vi "rqcBob Alice PM Level Test (Low Level Example).vi"() -> ()   [LabVIEW 2016]
uses:
  FPGA/rqcBob/Custom Controls/Pulse Train/rqcBob Pulse Train Config.ctl
  FPGA/rqcBob/Custom Controls/Pulse Train/rqcBob Pulse Train.Generation Mode.ctl
  FPGA/rqcBob/Custom Controls/Pulse Train/rqcBob Pulse Train.First Pulse Delay Mode.ctl
  FPGA/rqcBob/Custom Controls/rqcBob Window Config.ctl
  Shared/Shared FPGA Lib/Shared Logic/Custom Controls/rqc Random Generator.parameters.ctl
  Shared/Shared FPGA Lib/Shared Logic/Custom Controls/rqc Random Generator.value type.ctl
  FPGA/rqcBob/Custom Controls/rqcBob Modulator Config.ctl
  Custom Controls/rqcBob States.ctl
  FPGA/rqcBob/Custom Controls/rqcBob Trigger Type.ctl
  Shared/Shared Host Lib/rqc ServiceNET/Custom Controls/rqc ServiceNET command.ctl
  Shared/Shared Host Lib/rqc ServiceNET/Bob/Custom Controls/rqcBob ServiceNET control.ctl
  <vilib>/FPGAPlugInAG/PCIe-7841R/niLvFpga_Open_PCIe-7841R.vi
  <vilib>/rvi/interface/common/dynamic/niFpgaDynamicAddResources.vi
  Low Level API/Configuration/Photon Detector/Detection FIFOs config/rqcBob Configure PD Detect FIFO (1PD PD1).vi
  Low Level API/Configuration/Photon Detector/Set PD window/rqcBob Configure SPD Detection Window (1PD PD1).vi
  Low Level API/Read/Read PD Detection FIFO/rqcBob Read PD Detection FIFO (1PD PD1).vi
  Shared/Shared Host Lib/rqc ServiceNET/Bob/rqcBob Send Data/rqcBob ServiceNET Send Data U32.vi
  <vilib>/FPGAPlugInAG/Dynamic/niLvFpga_Close_Dynamic.vi
  <vilib>/rvi/interface/nirviOpenFPGA/nirviOpenFPGA.xnode
  FPGA Bitfiles/rqcBob (FPGA) 7841 v 2.1.0.lvbitx
  <vilib>/rvi/interface/nirviCloseFPGA/nirviCloseFPGA.xnode
panel:
  in  "modulator.clock delay":fxp<+,4,4>
  out "current States":T1=enum."App.Stop"
  out "error out":errorcluster
  out "Connected to Alice":bool
  in  "Stop":bool
  in  "modulator.config":T2={"modulator.start"=1200, "modulator.stop"=1500}
  in  "PD.detection window":u8=11
  in  "rndGen.parameters":T3={"value type"=enum."constant", "constant"=0, "num of levels"=0, "levels values"=[0, 0, 0, 0]}
  in  "window.config":T5={"window.open"=1340, "window.close"=1640}
  in  "train.configuration":T6={"train.period"=2000, "train.num of pulses"=300, "train.mode"=enum."train sequence.single", "train.num of trains"=2000, "train.first pulse delay mode"=enum."every train", "train.first pulse delay"=55}
  in  "Port:":u16=5020
  in  "Alice's IP address":string="192.168.0.228"
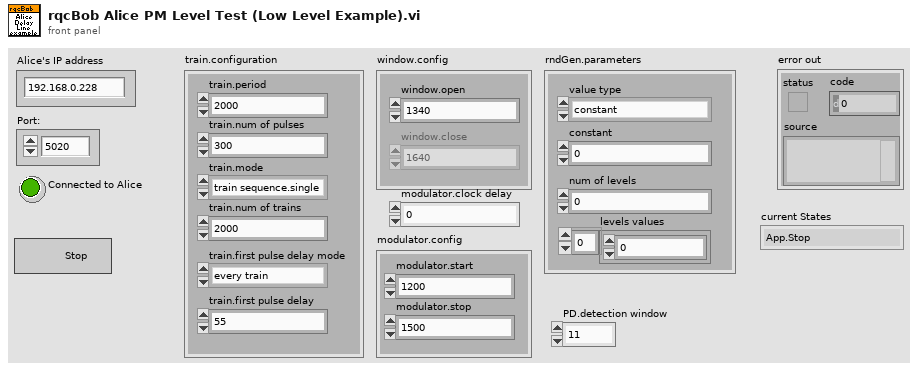
[diagram p1: front panel]
types:
  T1 = typedef "rqcBob States.ctl" = enum16{"HW.configure", "HW.sendTrigger", "HW.initiate", "HW.measure", "HW.stop", "NET.create", "NET.connect", "NET.sendCommand", "NET.readCommand", "NET.readData", "NET.close", "App.HandleEvent", "App.HandleError", "App.Stop"}
  T2 = typedef "rqcBob Modulator Config.ctl" = cluster{"modulator.start":u16, "modulator.stop":u16}
  T3 = typedef "rqc Random Generator.parameters.ctl" = cluster{"value type":T4, "constant":u16, "num of levels":u16, "levels values":u16[]}
  T4 = typedef "rqc Random Generator.value type.ctl" = enum16{"random value", "constant"}
  T5 = typedef "rqcBob Window Config.ctl" = cluster{"window.open":u16, "window.close":u16}
  T6 = typedef "rqcBob Pulse Train Config.ctl" = cluster{"train.period":u16, "train.num of pulses":u16, "train.mode":T7, "train.num of trains":u16, "train.first pulse delay mode":T8, "train.first pulse delay":u16}
  T7 = typedef "rqcBob Pulse Train.Generation Mode.ctl" = enum8{"single train", "train sequence.single", "train sequence.wait for trigger", "continuous"}
  T8 = typedef "rqcBob Pulse Train.First Pulse Delay Mode.ctl" = enum8{"none", "every train", "first train"}
  T9 = typedef "rqcBob Trigger Type.ctl" = enum16{"software", "immediate", "DIO"}
  T10 = typedef "rqc ServiceNET command.ctl" = enum8{"NONE", "READY", "START", "PING"}
  T11 = typedef "rqcBob ServiceNET control.ctl" = cluster{"connection ID":refnum<k5>, "connected?":bool, "Alice's IP address":string, "port":u16}
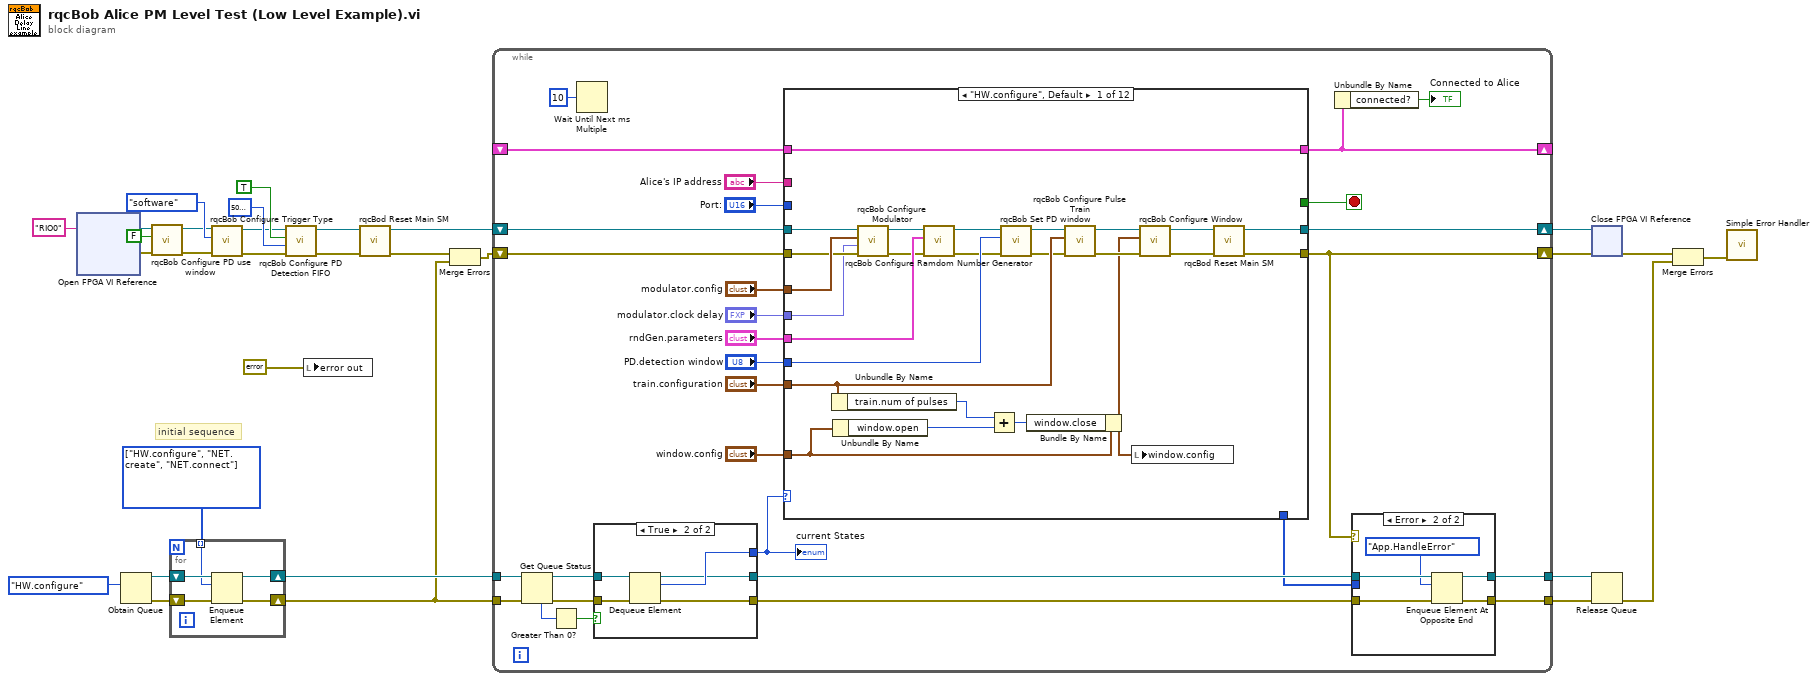
[diagram p0: block diagram]
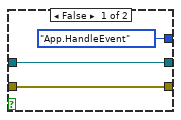
[diagram p2: hidden frame]
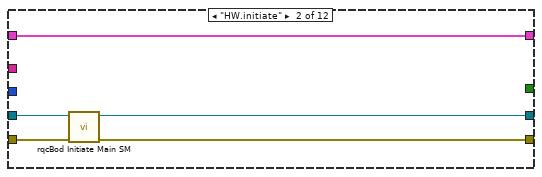
[diagram p3: hidden frame]
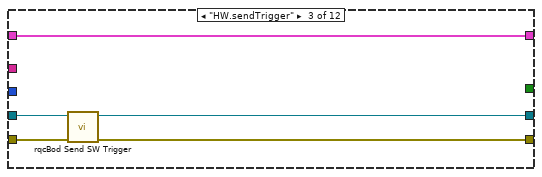
[diagram p4: hidden frame]
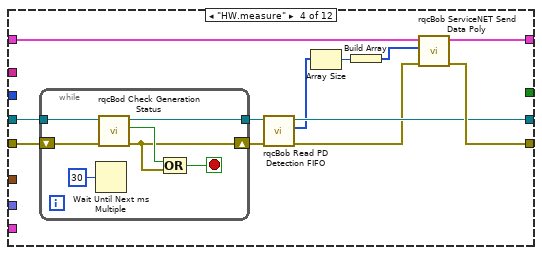
[diagram p5: hidden frame]
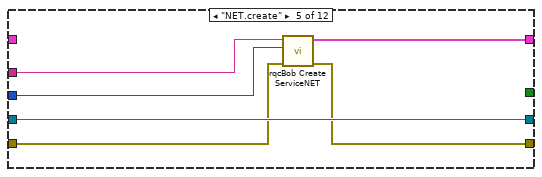
[diagram p6: hidden frame]
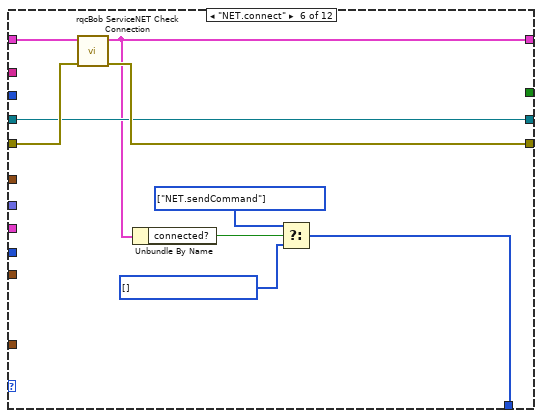
[diagram p7: hidden frame]
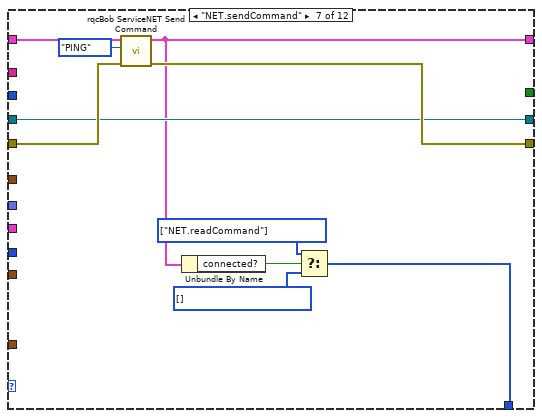
[diagram p8: hidden frame]
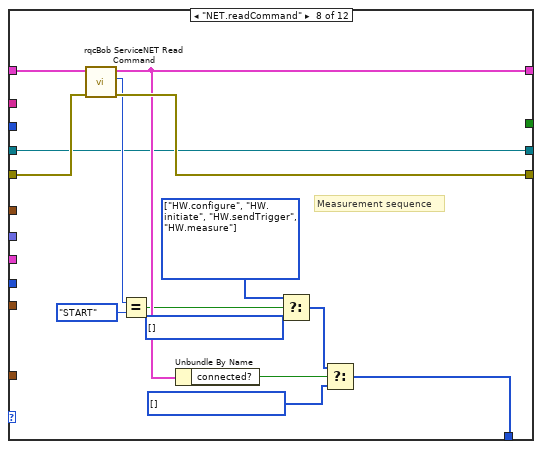
[diagram p9: hidden frame]
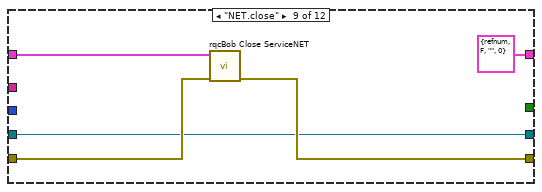
[diagram p10: hidden frame]
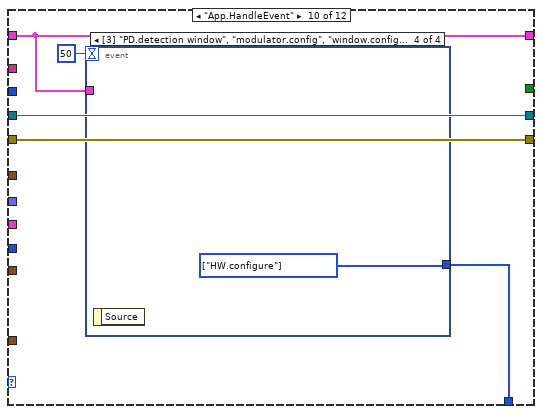
[diagram p11: hidden frame]
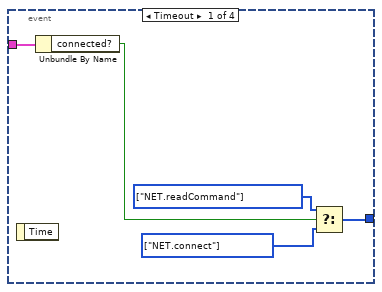
[diagram p12: hidden frame]
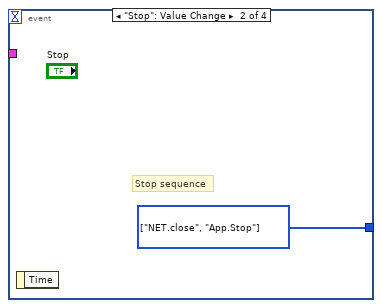
[diagram p13: hidden frame]
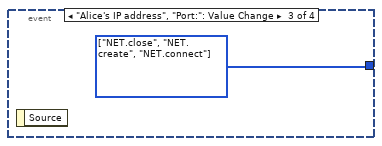
[diagram p14: hidden frame]
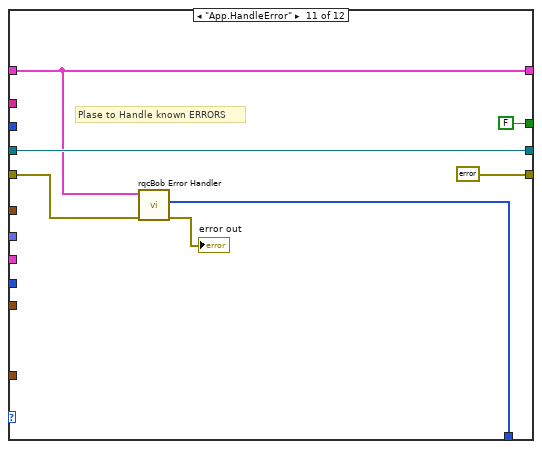
[diagram p15: hidden frame]
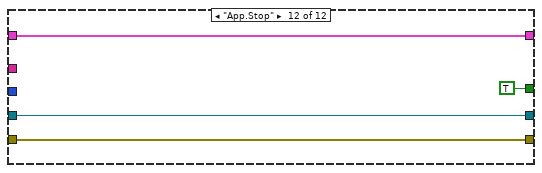
[diagram p16: hidden frame]
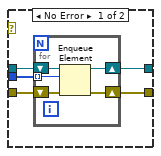
[diagram p17: hidden frame]
diagram:
  w21 = T1[] [enum."HW.configure", enum."NET.create", enum."NET.connect"] items=["HW.configure", "HW.sendTrigger", "HW.initiate", "HW.measure", "HW.stop", "NET.create", "NET.connect", "NET.sendCommand", "NET.readCommand", "NET.readData", "NET.close", "App.HandleEvent", "App.HandleError", "App.Stop"]
  # "initial sequence"
  n1 = xnode "Open FPGA VI Reference"("resource name"="RIO0") -> ("FPGA VI Reference Out"=w9:refnum<k20>, "error out"=w8:errorcluster)  [unwired: 1 in]
  n2 = Obtain Queue(element data type=rqcBob_States."HW.configure" ("rqcBob States")) -> (queue out=w26:refnum<queue>, error out=w25:errorcluster)  [unwired: 4 in, 1 out]
  n3 = call "rqcBob Configure PD use window.vi"("error in"=w8, "PD.use window"=FALSE ("SPD.use detector window"), "FPGA reference in"=w9) -> ("error out"=w27:errorcluster, "FPGA reference out"=w28:refnum<k20>)  [unwired: 7 in]
  n4 = for {
    tunnel: w21 -> [w31] mode=indexing
    shift-right: [w32] -> w23
    shift-left: w26 -> [w35]
    shift-right: [w33] -> w20
    shift-left: w25 -> [w34]
    n5 = Enqueue Element(queue=w35, element=w31, error in (no error)=w34) -> (queue out=w32:refnum<queue>, error out=w33:errorcluster)  [unwired: 1 in, 1 out]
  }
  n6 = call "rqcBob Configure Trigger Type.vi"("error in"=w27, "rqcBob Trigger Type"=rqcBob_Trigger_Type."software", "FPGA reference in"=w28) -> ("error out"=w1:errorcluster, "FPGA reference out"=w2:refnum<k20>)  [unwired: 7 in]
  n7 = call-poly "rqcBob Configure PD Detection FIFO.vi"("error in"=w1, "PD.detect fifo depth"=u32 5000000 ("SPD.detect fifo depth"), "PD.detect fifo write enable"=TRUE ("SPD.detect fifo write enable"), "FPGA reference in"=w2) -> ("error out"=w5:errorcluster, "FPGA reference out"=w6:refnum<k20>)  [unwired: 6 in]
  n8 = local write "error out"(errorcluster {"status"=FALSE, "code"=0, "source"=""} ("error constant")) -> ()
  n9 = call "rqcBod Reset Main SM.vi"("error in"=w5, "FPGA reference in"=w6) -> ("error out"=w10:errorcluster, "FPGA reference out"=w11:refnum<k20>)  [unwired: 8 in]
  n10 = Merge Errors(w10, w20) -> (w24:errorcluster)
  n11 = while {
    shift-right: [w45] -> w19
    shift-left: w24 -> [w56]
    shift-right: [w46] -> w18
    shift-left: w11 -> [w43]
    tunnel: w23 -> [w54]
    tunnel: w20 -> [w53]
    tunnel: [w48] -> w17
    tunnel: [w47] -> w16
    shift-right: [w39] -> _
    shift-left: _ -> [w40]
    stop <- w44 stop-if-true
    n12 = Get Queue Status(queue=w54, error in (no error)=w53) -> (queue out=w50:refnum<queue>, error out=w49:errorcluster, # elements in queue=w52:i32)  [unwired: 1 in, 5 out]
    n13 = Greater Than 0?(x=w52) -> (x > 0?=w51:bool)
    n14 = Wait Until Next ms Multiple(millisecond multiple=u32 10) -> ()  [unwired: 1 out]
    n15 = case shown="True" w51 {
      tunnel: w50 -> [w65 w72]
      tunnel: w49 -> [w66 w71]
      tunnel: [rqcBob_States."App.HandleEvent" ("rqcBob States") w70] -> w59
      tunnel: [w65 w69] -> w58
      tunnel: [w66 w68] -> w55
      frame False {
      }
      frame True {
        n16 = Dequeue Element(queue=w72, error in (no error)=w71) -> (queue out=w69:refnum<queue>, element=w70:T1, error out=w68:errorcluster)  [unwired: 1 in, 1 out]
      }
    }
    "current States" <- w59
    n17 = case shown="\"HW.configure\", Default" w59 {
      tunnel: "modulator.config" -> [w93 _ _ _ _ _ _ _ _ _ _ _]
      tunnel: "train.configuration" -> [w80 _ _ _ _ _ _ _ _ _ _ _]
      tunnel: "window.config" -> [w92 _ _ _ _ _ _ _ _ _ _ _]
      tunnel: "rndGen.parameters" -> [w91 _ _ _ _ _ _ _ _ _ _ _]
      tunnel: "PD.detection window" -> [w75 _ _ _ _ _ _ _ _ _ _ _]
      tunnel: [w82 w99 w104 w114 w127 w139 w149 w163 w167 w173 errorcluster {"status"=FALSE, "code"=0, "source"=""} ("error constant") w192] -> w45
      tunnel: w56 -> [w90 w101 w106 w118 w128 w140 w150 w164 w168 w173 w187 w192]
      tunnel: [_ _ _ _ _ w133 w142 w159 _ w172 w186 _] -> w57
      tunnel: [w84 w100 w105 w111 w132 w138 w148 w152 w166 w174 w189 w193] -> w46
      tunnel: [_ _ _ _ _ _ _ _ _ _ FALSE TRUE] -> w44
      tunnel: w43 -> [w89 w102 w107 w119 w132 w138 w148 w152 w166 w174 w189 w193]
      tunnel: "Alice's IP address" -> [_ _ _ _ w131 _ _ _ _ _ _ _]
      tunnel: "Port:" -> [_ _ _ _ w130 _ _ _ _ _ _ _]
      tunnel: [w81 w98 w103 w116 w129 w137 w146 w160 T11 {"connection ID"=refnum, "connected?"=FALSE, "Alice's IP address"="", "port"=0} ("rqcBob ServiceNET control") w171 w188 w191] -> w39
      tunnel: w40 -> [w81 w98 w103 w115 _ w141 w151 w165 w170 w171 w188 w191]
      tunnel: "modulator.clock delay" -> [w78 _ _ _ _ _ _ _ _ _ _ _]
      frame "HW.configure", Default {
        n18 = Unbundle By Name(w80) -> ("train.num of pulses"=w79:u16)
        n19 = Unbundle By Name(w92) -> ("window.open"=w97:u16)
        n20 = call "rqcBob Configure Modulator.vi"("error in"=w90, "modulator.clock delay"=w78, "modulator.config"=w93, "FPGA reference in"=w89) -> ("error out"=w88:errorcluster, "FPGA reference out"=w87:refnum<k20>)  [unwired: 6 in]
        n21 = call "rqcBob Configure Ramdom Number Generator.vi"("error in"=w88, "rqcBob rndGen.parameters"=w91, "FPGA reference in"=w87) -> ("error out"=w74:errorcluster, "FPGA reference out"=w76:refnum<k20>)  [unwired: 7 in]
        n22 = Add(x=w79, y=w97) -> (x+y=w94:u16)
        n23 = call-poly "rqcBob Set PD window.vi"("error in"=w74, "PD1.detection window"=w75, "FPGA reference in"=w76) -> ("error out"=w73:errorcluster, "FPGA reference out"=w77:refnum<k20>)  [unwired: 7 in]
        n24 = Bundle By Name(cluster=w92, "window.close"=w94) -> (w86:T5)
        n25 = call "rqcBob Configure Pulse Train.vi"("error in"=w73, "train.configuration"=w80, "FPGA reference in"=w77) -> ("error out"=w95:errorcluster, "FPGA reference out"=w96:refnum<k20>)  [unwired: 6 in, 1 out]
        n26 = local write "window.config"(w86) -> ()
        n27 = call "rqcBob Configure Window.vi"("error in"=w95, "window.config"=w86, "FPGA reference in"=w96) -> ("error out"=w83:errorcluster, "FPGA reference out"=w85:refnum<k20>)  [unwired: 7 in]
        n28 = call "rqcBod Reset Main SM.vi"("error in"=w83, "FPGA reference in"=w85) -> ("error out"=w82:errorcluster, "FPGA reference out"=w84:refnum<k20>)  [unwired: 8 in]
      }
      frame "HW.initiate" {
        n29 = call "rqcBod Initiate Main SM.vi"("error in"=w101, "FPGA reference in"=w102) -> ("error out"=w99:errorcluster, "FPGA reference out"=w100:refnum<k20>)  [unwired: 8 in]
      }
      frame "HW.sendTrigger" {
        n30 = call "rqcBod Send SW Trigger.vi"("error in"=w106, "FPGA reference in"=w107) -> ("error out"=w104:errorcluster, "FPGA reference out"=w105:refnum<k20>)  [unwired: 8 in]
      }
      frame "HW.measure" {
        n31 = while {
          tunnel: w119 -> [w126]
          shift-right: [w120] -> w108
          shift-left: w118 -> [w125]
          tunnel: [w122] -> w112
          stop <- w121 stop-if-true
          n32 = Wait Until Next ms Multiple(millisecond multiple=u32 30) -> ()  [unwired: 1 out]
          n33 = call "rqcBod Check Generation Status.vi"("error in"=w125, "FPGA reference in"=w126) -> ("error out"=w120:errorcluster, "generation.done"=w123:bool, "FPGA reference out"=w122:refnum<k20>)  [unwired: 7 in]
          n34 = Compound Arithmetic op=OR(w123, w120) -> (w121:bool)
        }
        n35 = call-poly "rqcBob Read PD Detection FIFO.vi"("error in"=w108, "FPGA reference in"=w112) -> ("error out"=w109:errorcluster, "Data"=w110:u32[], "FPGA reference out"=w111:refnum<k20>)  [unwired: 6 in, 1 out]
        n36 = Array Size(array=w110) -> (size(s)=w117:i32)
        n37 = Build Array(w117) -> (w113:i32[])
        n38 = call-poly "rqcBob ServiceNET Send Data Poly.vi"("error in"=w109, "Data"=w113, "rqcBob ServiceNET in"=w115) -> ("error out"=w114:errorcluster, "rqcBob ServiceNET out"=w116:T11)  [unwired: 7 in]
      }
      frame "NET.create" {
        n39 = call "rqcBob Create ServiceNET.vi"("error in"=w128, "port"=w130, "Alice's IP address"=w131) -> ("error out"=w127:errorcluster, "rqcBob ServiceNET control"=w129:T11)  [unwired: 7 in]
      }
      frame "NET.connect" {
        w134 = T1[] [] items=["HW.configure", "HW.sendTrigger", "HW.initiate", "HW.measure", "HW.stop", "NET.create", "NET.connect", "NET.sendCommand", "NET.readCommand", "NET.readData", "NET.close", "App.HandleEvent", "App.HandleError", "App.Stop"] ("f")
        w136 = T1[] [enum."NET.sendCommand"] items=["HW.configure", "HW.sendTrigger", "HW.initiate", "HW.measure", "HW.stop", "NET.create", "NET.connect", "NET.sendCommand", "NET.readCommand", "NET.readData", "NET.close", "App.HandleEvent", "App.HandleError", "App.Stop"]
        n40 = call "rqcBob ServiceNET Check Connection.vi"("error in"=w140, "rqcBob ServiceNET in"=w141) -> ("error out"=w139:errorcluster, "rqcBob ServiceNET out"=w137:T11)  [unwired: 8 in]
        n41 = Unbundle By Name(w137) -> ("connected?"=w135:bool)
        n42 = Select(t=w136, s=w135, f=w134) -> (s? t:f=w133:T1[])
      }
      frame "NET.sendCommand" {
        w143 = T1[] [] items=["HW.configure", "HW.sendTrigger", "HW.initiate", "HW.measure", "HW.stop", "NET.create", "NET.connect", "NET.sendCommand", "NET.readCommand", "NET.readData", "NET.close", "App.HandleEvent", "App.HandleError", "App.Stop"] ("f")
        w144 = T1[] [enum."NET.readCommand"] items=["HW.configure", "HW.sendTrigger", "HW.initiate", "HW.measure", "HW.stop", "NET.create", "NET.connect", "NET.sendCommand", "NET.readCommand", "NET.readData", "NET.close", "App.HandleEvent", "App.HandleError", "App.Stop"] ("f")
        n43 = call "rqcBob ServiceNET Send Command.vi"("error in"=w150, "command"=rqc_ServiceNET_command."PING", "rqcBob ServiceNET in"=w151) -> ("error out"=w149:errorcluster, "rqcBob ServiceNET out"=w146:T11)  [unwired: 7 in]
        n44 = Unbundle By Name(w146) -> ("connected?"=w145:bool)
        n45 = Select(t=w144, s=w145, f=w143) -> (s? t:f=w142:T1[])
      }
      frame "NET.readCommand" {
        w154 = T1[] [] items=["HW.configure", "HW.sendTrigger", "HW.initiate", "HW.measure", "HW.stop", "NET.create", "NET.connect", "NET.sendCommand", "NET.readCommand", "NET.readData", "NET.close", "App.HandleEvent", "App.HandleError", "App.Stop"] ("f")
        w161 = T1[] [] items=["HW.configure", "HW.sendTrigger", "HW.initiate", "HW.measure", "HW.stop", "NET.create", "NET.connect", "NET.sendCommand", "NET.readCommand", "NET.readData", "NET.close", "App.HandleEvent", "App.HandleError", "App.Stop"] ("f")
        w155 = T1[] [enum."HW.configure", enum."HW.initiate", enum."HW.sendTrigger", enum."HW.measure"] items=["HW.configure", "HW.sendTrigger", "HW.initiate", "HW.measure", "HW.stop", "NET.create", "NET.connect", "NET.sendCommand", "NET.readCommand", "NET.readData", "NET.close", "App.HandleEvent", "App.HandleError", "App.Stop"] ("f")
        # "Measurement sequence"
        n46 = call "rqcBob ServiceNET Read Command.vi"("error in"=w164, "rqcBob ServiceNET in"=w165) -> ("error out"=w163:errorcluster, "command"=w158:T10, "rqcBob ServiceNET out"=w160:T11)  [unwired: 6 in, 1 out]
        n47 = Equal?(x=w158, y=rqc_ServiceNET_command."START") -> (x = y?=w156:bool)
        n48 = Unbundle By Name(w160) -> ("connected?"=w162:bool)
        n49 = Select(t=w155, s=w156, f=w154) -> (s? t:f=w153:T1[])
        n50 = Select(t=w153, s=w162, f=w161) -> (s? t:f=w159:T1[])
      }
      frame "NET.close" {
        n51 = call "rqcBob Close ServiceNET.vi"("error in"=w168, "rqcBob ServiceNET control"=w170) -> ("error out"=w167:errorcluster)  [unwired: 9 in]
      }
      frame "App.HandleEvent" {
        n52 = event shown="[3] \"PD.detection window\", \"modulator.config\", \"window.config\", \"rndGen.parameters.value type\", \"rndGen.parameters.num of levels\", \"rndGen.parameters.levels values\", \"rndGen.parameters\": Value Change" {
          selector: _ -> [_ _ _ _]
          dyn-events: _ -> [_ _ _ _]
          timeout: 50 -> [_ _ _ _]
          tunnel: [w179 w181 w182 w183] -> w172
          tunnel: w171 -> [w180 _ _ _]
          event Timeout {
            w176 = T1[] [enum."NET.connect"] items=["HW.configure", "HW.sendTrigger", "HW.initiate", "HW.measure", "HW.stop", "NET.create", "NET.connect", "NET.sendCommand", "NET.readCommand", "NET.readData", "NET.close", "App.HandleEvent", "App.HandleError", "App.Stop"]
            w177 = T1[] [enum."NET.readCommand"] items=["HW.configure", "HW.sendTrigger", "HW.initiate", "HW.measure", "HW.stop", "NET.create", "NET.connect", "NET.sendCommand", "NET.readCommand", "NET.readData", "NET.close", "App.HandleEvent", "App.HandleError", "App.Stop"]
            n53 = event-data() -> ()  [unwired: 1 in, 1 out]
            n54 = Unbundle By Name(w180) -> ("connected?"=w178:bool)
            n55 = Select(t=w177, s=w178, f=w176) -> (s? t:f=w179:T1[])
          }
          event "Stop": Value Change {
            w181 = T1[] [enum."NET.close", enum."App.Stop"] items=["HW.configure", "HW.sendTrigger", "HW.initiate", "HW.measure", "HW.stop", "NET.create", "NET.connect", "NET.sendCommand", "NET.readCommand", "NET.readData", "NET.close", "App.HandleEvent", "App.HandleError", "App.Stop"]
            # "Stop sequence"
            n56 = event-data() -> ()  [unwired: 1 in, 1 out]
          }
          event "Alice's IP address", "Port:": Value Change {
            w182 = T1[] [enum."NET.close", enum."NET.create", enum."NET.connect"] items=["HW.configure", "HW.sendTrigger", "HW.initiate", "HW.measure", "HW.stop", "NET.create", "NET.connect", "NET.sendCommand", "NET.readCommand", "NET.readData", "NET.close", "App.HandleEvent", "App.HandleError", "App.Stop"]
            n57 = event-data() -> ()  [unwired: 1 in, 1 out]
          }
          event "PD.detection window": Value Change {
            w183 = T1[] [enum."HW.configure"] items=["HW.configure", "HW.sendTrigger", "HW.initiate", "HW.measure", "HW.stop", "NET.create", "NET.connect", "NET.sendCommand", "NET.readCommand", "NET.readData", "NET.close", "App.HandleEvent", "App.HandleError", "App.Stop"]
            n58 = event-data() -> ()  [unwired: 1 in, 1 out]
          }
        }
      }
      frame "App.HandleError" {
        # "Plase to Handle known ERRORS"
        n59 = call "rqcBob Error Handler.vi"("error in (no error)"=w187, "rqcBob ServiceNET control"=w188) -> ("error out"=→"error out":errorcluster, "error sequence"=w186:T1[])  [unwired: 8 in]
      }
      frame "App.Stop" {
      }
    }
    n60 = Unbundle By Name(w39) -> ("connected?"=→"Connected to Alice":bool)
    n61 = case shown="Error" w45 {
      tunnel: w58 -> [w199 w209]
      tunnel: w57 -> [w196 _]
      tunnel: w55 -> [w195 w208]
      tunnel: [w198 w206] -> w48
      tunnel: [w197 w205] -> w47
      frame No Error {
        n62 = for {
          tunnel: w196 -> [w203] mode=indexing
          shift-right: [w201] -> w197
          shift-left: w195 -> [w202]
          shift-right: [w200] -> w198
          shift-left: w199 -> [w204]
          n63 = Enqueue Element(queue=w204, element=w203, error in (no error)=w202) -> (queue out=w200:refnum<queue>, error out=w201:errorcluster)  [unwired: 1 in, 1 out]
        }
      }
      frame Error {
        n64 = Enqueue Element At Opposite End(queue=w209, element=rqcBob_States."App.HandleError", error in (no error)=w208) -> (queue out=w206:refnum<queue>, error out=w205:errorcluster)  [unwired: 1 in, 1 out]
      }
    }
  }
  n65 = xnode "Close FPGA VI Reference"("FPGA VI Reference In"=w18, "error in"=w19) -> ("error out"=w15:errorcluster)
  n66 = Release Queue(queue=w17, error in (no error)=w16) -> (error out=w14:errorcluster)  [unwired: 1 in, 2 out]
  n67 = Merge Errors(w15, w14) -> (w13:errorcluster)
  n68 = call <vilib>:"Simple Error Handler.vi"("error in (no error)"=w13) -> ()  [unwired: 4 in, 5 out]
